vi "Test 7 zoneight234 to z1ight234.vi"(8 "error in (no error)":errorcluster, 11 "Test Case In":refnum<class "Descrambler Test.lvclass">) -> (0 "error out":errorcluster, 3 "Test Case Out":refnum<class "Descrambler Test.lvclass">)   [LabVIEW 2020, in "Descrambler Test.lvclass"]
uses:
  Descrambler Test.lvclass
  Descrambler Test.lvclass/Descrambler Test.ctl
  4993e8ee-a06a-463a-9684-69129f64d5ce.vi
  Words to Numbers Converter/Words to Numbers Converter.lvclass
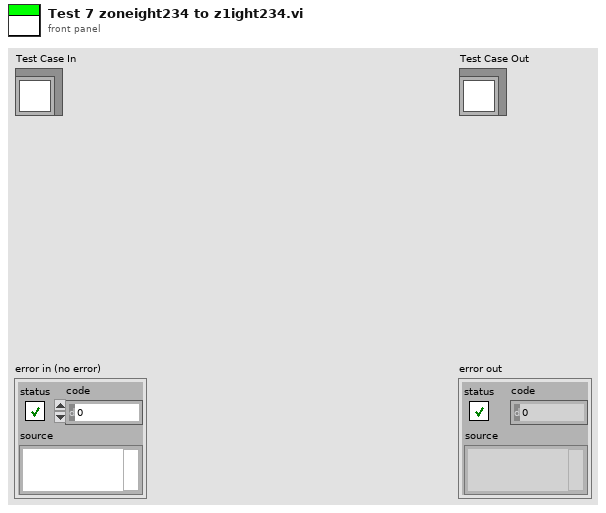
[diagram p1: front panel]
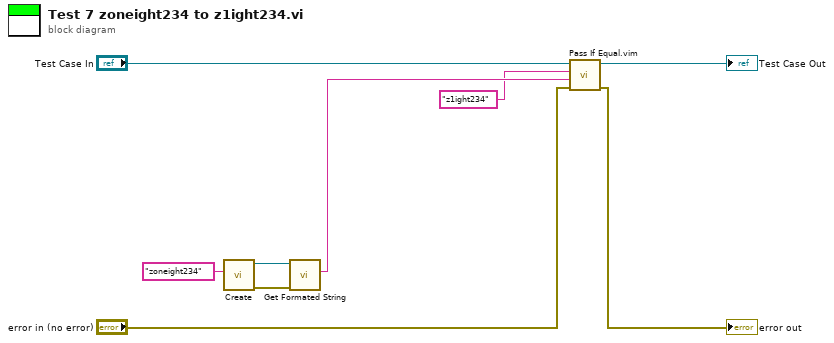
[diagram p0: block diagram]
diagram:
  n1 = call "Create.vi"("String"="zoneight234") -> ("error out"=w4:errorcluster, "Words to Numbers Converter"=w5:refnum<class "Words to Numbers Converter.lvclass">)  [unwired: 9 in]
  n2 = call "Get Formated String.vi"("error in (no error)"=w4, "Words to Numbers Converter in"=w5) -> ("String"=w2:string)  [unwired: 7 in, 2 out]
  n3 = call "Pass If Equal.vim"("error in (no error)"="error in (no error)", "Actual"=w2, "Expected"="z1ight234" ("String"), "LUnit Test Case In"="Test Case In") -> ("error out"=→"error out":errorcluster, "LUnit Test Case Out"=→"Test Case Out":refnum<class "Descrambler Test.lvclass">)  [unwired: 6 in]
